vi "Write Channel Setting.vi"(8 "error in (no error)":errorcluster, 10 "Channel Setting":T1, 11 "KH7008 in":refnum<class "Instrument.KH7008.lvclass">) -> (0 "error out":errorcluster, 3 "KH7008 out":refnum<class "Instrument.KH7008.lvclass">)   [LabVIEW 2016, in "Instrument.KH7008.lvclass"]
uses:
  Instrument.KH7008.lvclass
  typedefs/KH_control_array.ctl
  typedefs/KH_control.ctl
  typedefs/Channel-Enum.ctl
  typedefs/Gain-Enum.ctl
  typedefs/Shunt-Enum.ctl
  typedefs/Input Configuration-Enum.ctl
  Instrument.KH7008.lvclass/Instrument.KH7008.ctl
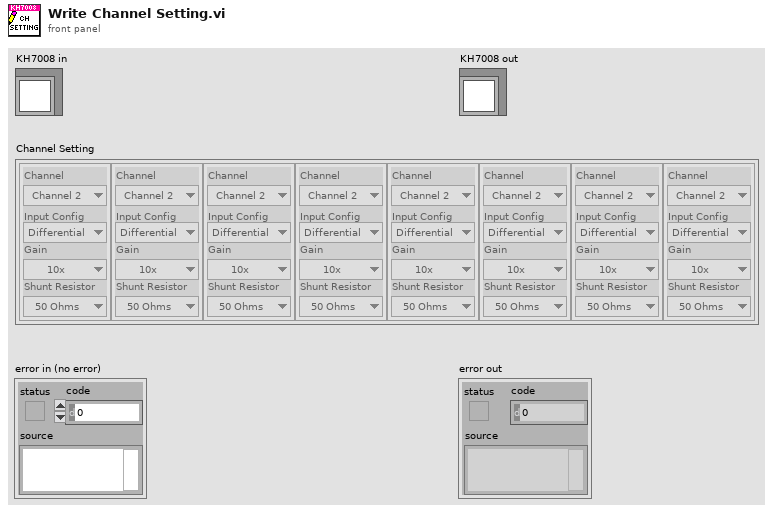
[diagram p1: front panel]
types:
  T1 = typedef "Instrument.KH7008.lvclass/KH_control_array.ctl" = T2[]
  T2 = typedef "Instrument.KH7008.lvclass/KH_control.ctl" = cluster{"Channel":T3, "Gain":T4, "Shunt Resistor":T5, "Input Config":T6}
  T3 = typedef "Instrument.KH7008.lvclass/Channel-Enum.ctl" = enum16{"Channel 1", "Channel 2", "Channel 3", "Channel 4", "Channel 5", "Channel 6", "Channel 7", "Channel 8"}
  T4 = typedef "Instrument.KH7008.lvclass/Gain-Enum.ctl" = enum16{"1x", "10x", "100x", "1000x"}
  T5 = typedef "Instrument.KH7008.lvclass/Shunt-Enum.ctl" = enum16{"Open", "50 Ohms", "500 Ohms", "5k Ohms", "50k Ohms"}
  T6 = typedef "Instrument.KH7008.lvclass/Input Configuration-Enum.ctl" = enum16{"Ground", "SE+ (-gnd)", "SE- (+gnd)", "Differential"}
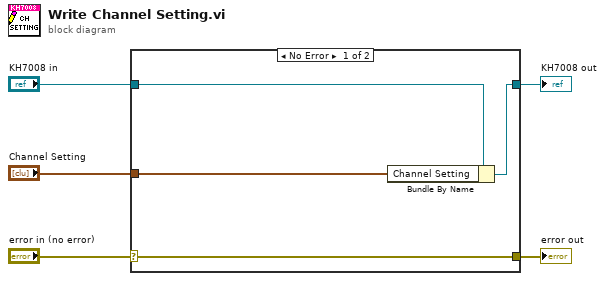
[diagram p0: block diagram]
diagram:
  n1 = case shown="No Error" "error in (no error)" {
    selector: "error in (no error)" -> [w9 w10]
    tunnel: [w9 w10] -> w4
    tunnel: [w7 w11] -> w2
    tunnel: "KH7008 in" -> [w8 w11]
    tunnel: "Channel Setting" -> [w6 _]
    frame No Error {
      n2 = Bundle By Name(cluster=w8, "Channel Setting"=w6) -> (w7:refnum<class "Instrument.KH7008.lvclass">)
    }
    frame Error {
    }
  }
  "error out" <- w4
  "KH7008 out" <- w2
